vi "Set Array of Conflict Zones.vi"(8 "error in (no error)":errorcluster, 10 "Array of Conflict Zones":T1[](array[typedef]) caption="Conflict Zones (unit in mm)", 11 "VacuumLines Configuration in":refnum<class "VacuumLines Configuration.lvclass">) -> (0 "error out":errorcluster, 3 "VacuumLines Configuration out":refnum<class "VacuumLines Configuration.lvclass">)   [LabVIEW 2016, in "Hardware.lvlib" / "VacuumLine.lvlib" / "VacuumLines Configuration.lvclass"]
uses:
  <userlib>/Common Components/Hardware/Abstract System/VacuumLine/VacuumLines Configuration/VacuumLines Configuration.lvclass
  <userlib>/Common Components/Hardware/Abstract System/VacuumLine/VacuumLines/Conflict Zone.ctl
  <userlib>/Common Components/Hardware/Abstract System/VacuumLine/VacuumLines Configuration/VacuumLines Configuration.lvclass/VacuumLines Configuration.ctl
  <userlib>/Common Components/Hardware/Abstract System/VacuumLine/VacuumLines/VacuumLines.lvclass/VacuumLines.ctl
  <userlib>/Common Components/Hardware/Abstract System/VacuumLine/VacuumLines/VacuumLines.lvclass
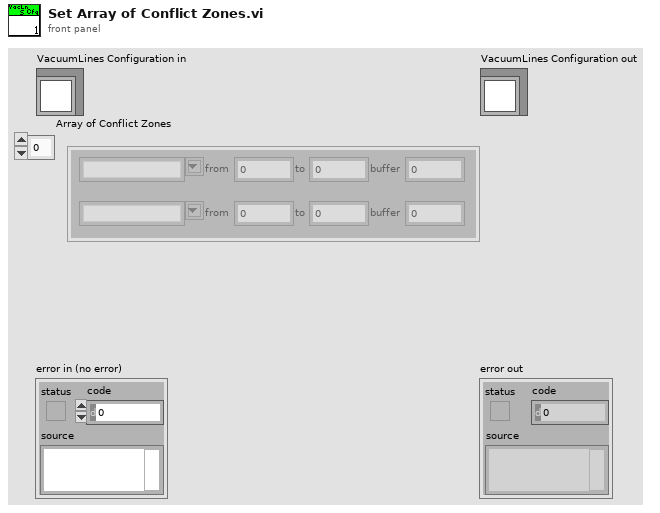
[diagram p1: front panel]
types:
  T1 = typedef "Hardware.lvlib/VacuumLine.lvlib/VacuumLines.lvclass/Conflict Zone.ctl" = cluster{"Conflict Zone":cluster{"1":cluster{"Label":string, "from":dbl, "to":dbl, "buffer":dbl}, "2":cluster{"Label":string, "from":dbl, "to":dbl, "buffer":dbl}}}
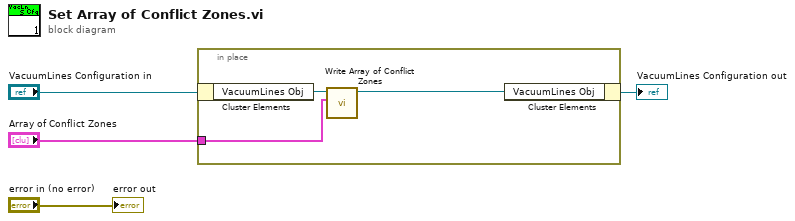
[diagram p0: block diagram]
diagram:
  n1 = in-place {
    in-place-border: "Array of Conflict Zones" -> [w5]
    n2 = in-place-cluster #1("VacuumLines Configuration in") -> ("VacuumLines Obj"=w7:refnum<class "VacuumLines.lvclass">)
    n3 = call <userlib>:"Write Array of Conflict Zones.vi"("Array of Conflict Zones"=w5, "VacuumLines in"=w7) -> ("VacuumLines out"=w6:refnum<class "VacuumLines.lvclass">)  [unwired: 9 in]
    n4 = in-place-cluster #1("VacuumLines Obj"=w6) -> (→"VacuumLines Configuration out":refnum<class "VacuumLines Configuration.lvclass">)
  }
  "error out" <- "error in (no error)"
